vi "Test Queue Synch.vi"() -> ()   [LabVIEW 2021]
uses:
  Source/Support/Nodes/abs_Node/Status.ctl
  Source/System/bt_System.lvclass
  Source/Support/Nodes/Decorators/Repeater/Support/Finish On - Type.ctl
  Source/Support/Nodes/Composites/abs_Parallel/Support/Status Calculation.ctl
  Source/Blackboard/Blackboard.lvclass
  Source/Blackboard/Blackboard.lvclass/Blackboard.ctl
  Source/Support/Nodes/Leaves/abs_Type Leaf/abs_Type Leaf.lvclass/abs_Type Leaf.ctl
  Source/Blackboard/Get Value Type/Get Boolean.vi
  Source/Blackboard/Get Value Type/Get String.vi
  Source/Blackboard/Get Value Type/Get I32.vi
  <vilib>/TSA/Abstract Data Classes/Abs_Types/String/Static Read.vi
  <vilib>/TSA/Abstract Data Classes/Abs_Types/I32 Integer/Static Read.vi
  <vilib>/TSA/Abstract Data Classes/Abs_Types/Boolean/Static Read.vi
  Source/Blackboard/Support/Index Group.vi
  Source/Blackboard/Support/Index Tags.vi
  Source/Support/Nodes/Leaves/abs_Type Leaf/Properties/Write Value Class.vi
  <vilib>/TSA/Omni-Bus/Local Bus/Support/Bool/Local Bus_Boolean.lvclass
  C:/Program Files (x86)/National Instruments/LabVIEW 2021/vi.lib/TSA/Abstract Data Classes/Abs_Types/Value/Abs_Value.lvclass
  Source/Support/Nodes/Leaves/Test Boolean/Test Abs_Boolean.lvclass
  C:/Users/Tim/Documents/GitHub/LV_Behaviour_Tree/Source/Support/Nodes/abs_Node/bt_Node.lvclass
  C:/Users/Tim/Documents/GitHub/LV_Behaviour_Tree/Source/Support/Nodes/Leaves/abs_Type Leaf/abs_Type Leaf.lvclass
  <vilib>/TSA/Abstract Data Classes/Abs_Types/Boolean/Abs_Boolean.lvclass
  C:/Program Files (x86)/National Instruments/LabVIEW 2021/vi.lib/TSA/Abstract Data Classes/Abs_Types/Type/Abs_Type.lvclass
  <vilib>/TSA/Omni-Bus/Local Bus/Support/I32/Local Bus_I32.lvclass
  <vilib>/TSA/Omni-Bus/Local Bus/Support/STR/Local Bus_String.lvclass
  Source/Support/Nodes/Leaves/Synch/Queue/Send/bt_Send_Queue.lvclass
  Source/Support/Nodes/Leaves/Synch/Queue/WaitOn/bt_WaitOn_Queue.lvclass
  <vilib>/TSA/Omni-Bus/Local Bus/Support/Initialise DVR's.vi
  <vilib>/TSA/Abstract Data Classes/Abs_Types/Value/Abs_Value.lvclass
  <vilib>/TSA/Abstract Data Classes/Abs_Types/Type/Abs_Type.lvclass
  <vilib>/TSA/Omni-Bus/Local Bus/Support/DBL/Local Bus_DBL.lvclass
  <vilib>/TSA/Omni-Bus/Local Bus/Support/SGL/Local Bus_SGL.lvclass
  <vilib>/TSA/Omni-Bus/Local Bus/Support/EXT/Local Bus_EXT.lvclass
  <vilib>/TSA/Omni-Bus/Local Bus/Support/Variant/Local Bus_Variant.lvclass
  <vilib>/TSA/Omni-Bus/Local Bus/Support/WFM/Local Bus_Waveform.lvclass
  <vilib>/TSA/Omni-Bus/Local Bus/Support/Time/Local Bus_Time.lvclass
  <vilib>/TSA/Omni-Bus/Local Bus/Support/U8/Local Bus_U8.lvclass
  <vilib>/TSA/Omni-Bus/Local Bus/Support/U16/Local Bus_U16.lvclass
  <vilib>/TSA/Omni-Bus/Local Bus/Support/U32/Local Bus_U32.lvclass
  <vilib>/TSA/Omni-Bus/Local Bus/Support/U64/Local Bus_U64.lvclass
  <vilib>/TSA/Omni-Bus/Local Bus/Support/I8/Local Bus_I8.lvclass
  <vilib>/TSA/Omni-Bus/Local Bus/Support/I16/Local Bus_I16.lvclass
  <vilib>/TSA/Omni-Bus/Local Bus/Support/I64/Local Bus_I64.lvclass
  <vilib>/TSA/Omni-Bus/Local Bus/Support/CSGL/Local Bus_CSGL.lvclass
  <vilib>/TSA/Omni-Bus/Local Bus/Support/CDBL/Local Bus_CDBL.lvclass
  <vilib>/TSA/Omni-Bus/Local Bus/Support/CEXT/Local Bus_CEXT.lvclass
  <vilib>/TSA/Omni-Bus/Local Bus/Support/Type/Local Bus_Type.lvclass
  <vilib>/TSA/Abstract Data Classes/Abs_Types/I32 Integer/Abs_I32 Integer.lvclass
  <vilib>/TSA/Abstract Data Classes/Abs_Types/String/Abs_String.lvclass
  Source/BT.lvlib
  Source/Support/Nodes/Composites/abs_Parallel/bt_Parallel.lvclass
  Source/Support/Nodes/Decorators/Repeater/bt_Repeater.lvclass
  Source/Support/Nodes/abs_Node/bt_Node.lvclass
panel:
  out "error out 4":errorcluster
  out "error out 3":errorcluster
  out "error out 2":errorcluster
  out "error out":errorcluster
  out "String":string
  out "Value":i32
  out "Boolean":bool
  in  "stop":bool
  out "Status":T1
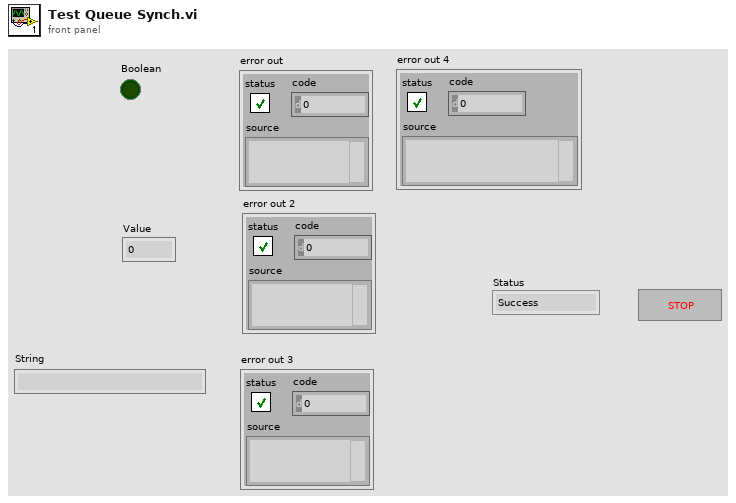
[diagram p1: front panel]
types:
  T1 = typedef "BT.lvlib/bt_Node.lvclass/Status.ctl" = enum16{"Success", "Failure", "Running"}
  T2 = typedef "BT.lvlib/bt_Parallel.lvclass/Status Calculation.ctl" = enum16{"Succeed on All Succeed", "Failure on All Failure", "Succeed on Any Succeed", "Failure on Any Failure"}
  T3 = typedef "BT.lvlib/bt_Repeater.lvclass/Finish On - Type.ctl" = enum16{"Success", "Failure", "Never"}
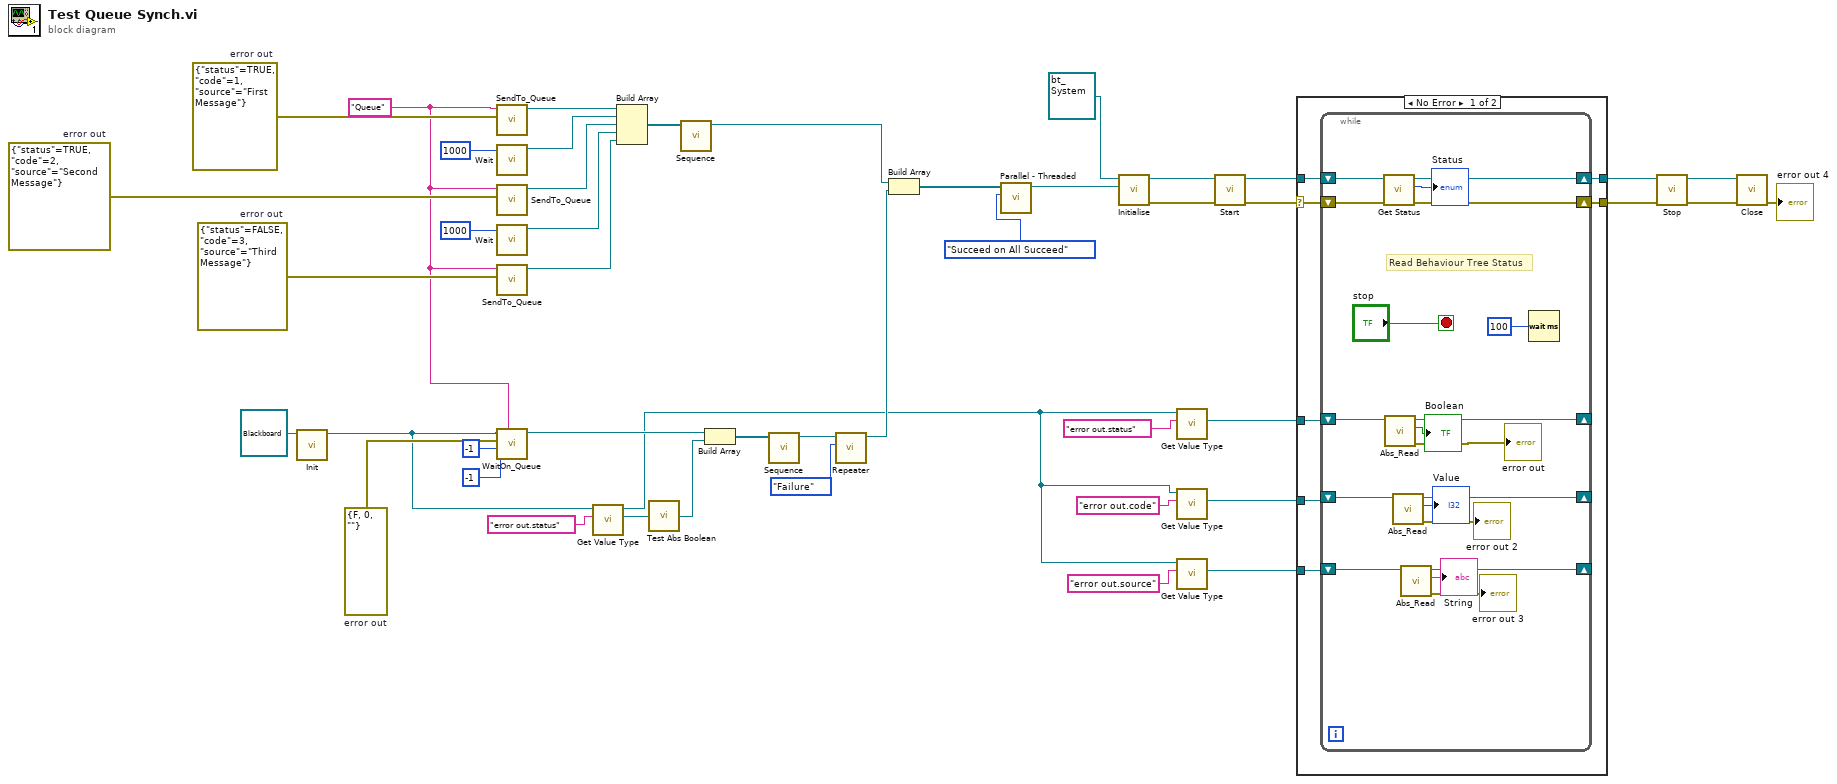
[diagram p0: block diagram]
diagram:
  w16 = errorcluster {"status"=FALSE, "code"=3, "source"="Third Message"}  # error out
  w18 = errorcluster {"status"=TRUE, "code"=2, "source"="Second Message"}  # error out
  w19 = errorcluster {"status"=TRUE, "code"=1, "source"="First Message"}  # error out
  w20 = errorcluster {"status"=FALSE, "code"=0, "source"=""}  # error out
  w6 = "Queue" ("Name")
  n1 = call-dynamic "Init.vi"("bt_Blackboard in"=refnum<class "Blackboard.lvclass"> refnum) -> ("bt_Blackboard out"=w11:refnum<class "Blackboard.lvclass">)  [unwired: 9 in, 1 out]
  n2 = call "SendTo_Queue.vi"("Message"=w19, "Queue Name"=w6) -> ("Queue Out"=w35:refnum<class "bt_Send_Queue.lvclass">)  [unwired: 9 in]
  n3 = call "Wait.vi"("Time (ms)"=u32 1000) -> ("Node Out"=w27:refnum<class "bt_Node.lvclass">)  [unwired: 10 in]
  n4 = call "SendTo_Queue.vi"("Message"=w18, "Queue Name"=w6) -> ("Queue Out"=w33:refnum<class "bt_Send_Queue.lvclass">)  [unwired: 9 in]
  n5 = call "Wait.vi"("Time (ms)"=u32 1000) -> ("Node Out"=w25:refnum<class "bt_Node.lvclass">)  [unwired: 10 in]
  n6 = call "SendTo_Queue.vi"("Message"=w16, "Queue Name"=w6) -> ("Queue Out"=w32:refnum<class "bt_Send_Queue.lvclass">)  [unwired: 9 in]
  n7 = call "WaitOn_Queue.vi"("Queue Name"=w6, "Max Queue Size"=-1, "Timeout (ms)"=-1, "Message Type"=w20, "bt_Blackboard in"=w11) -> ("Queue out"=w30:refnum<class "bt_WaitOn_Queue.lvclass">)  [unwired: 5 in, 1 out]
  n8 = call-poly "Get Value Type.vi"("Tag"="error out.status", "Blackboard in"=w11) -> ("Value"=w12:refnum<class "Abs_Boolean.lvclass">, "Blackboard out"=w5:refnum<class "Blackboard.lvclass">)  [unwired: 6 in, 2 out]
  n9 = Build Array(w35, w27, w33, w25, w32) -> (w34:refnum<class "bt_Node.lvclass">[])
  n10 = call "Test Abs Boolean.vi"("Abs_Boolean.lvclass"=w12) -> ("abs_Node"=w24:refnum<class "bt_Node.lvclass">)  [unwired: 4 in]
  n11 = call "Sequence.vi"("Nodes"=w34) -> ("Node"=w31:refnum<class "bt_Node.lvclass">)  [unwired: 10 in]
  n12 = Build Array(w30, w24) -> (w29:refnum<class "bt_Node.lvclass">[])
  n13 = call "Sequence.vi"("Nodes"=w29) -> ("Node"=w23:refnum<class "bt_Node.lvclass">)  [unwired: 10 in]
  n14 = call "Repeater.vi"("Finish On"=Finish_On_-_Type."Failure", "Node In"=w23) -> ("Node Out"=w21:refnum<class "bt_Node.lvclass">)  [unwired: 9 in]
  n15 = Build Array(w31, w21) -> (w37:refnum<class "bt_Node.lvclass">[])
  n16 = call "Parallel - Threaded.vi"("Status Calculation"=Status_Calculation."Succeed on All Succeed", "Nodes"=w37) -> ("Node"=w36:refnum<class "bt_Node.lvclass">)  [unwired: 9 in]
  n17 = call "Initialise.vi"("Behaviour Tree"=w36, "bt_System in"=refnum<class "bt_System.lvclass"> refnum) -> ("error out"=w45:errorcluster, "bt_System out"=w46:refnum<class "bt_System.lvclass">)  [unwired: 8 in]
  n18 = call-poly "Get Value Type.vi"("Tag"="error out.status", "Blackboard in"=w5) -> ("Value"=w14:refnum<class "Abs_Boolean.lvclass">)  [unwired: 6 in, 3 out]
  n19 = call-poly "Get Value Type.vi"("Tag"="error out.code", "Blackboard in"=w5) -> ("Value"=w8:refnum<class "Abs_I32 Integer.lvclass">)  [unwired: 6 in, 3 out]
  n20 = call-poly "Get Value Type.vi"("Tag"="error out.source", "Blackboard in"=w5) -> ("Value"=w4:refnum<class "Abs_String.lvclass">)  [unwired: 6 in, 3 out]
  n21 = call "Start.vi"("error in (no error)"=w45, "bt_System in"=w46) -> ("error out"=w3:errorcluster, "bt_System out"=w43:refnum<class "bt_System.lvclass">)  [unwired: 8 in]
  n22 = case shown="No Error" w3 {
    selector: w3 -> [w48 w73]
    tunnel: w43 -> [w53 w74]
    tunnel: [w52 w74] -> w40
    tunnel: w14 -> [w51 _]
    tunnel: w8 -> [w50 _]
    tunnel: w4 -> [w49 _]
    tunnel: [w47 w73] -> w2
    frame No Error {
      n23 = while {
        shift-right: [w70] -> w52
        shift-left: w53 -> [w71]
        shift-right: [w66] -> _
        shift-left: w51 -> [w67]
        shift-right: [w64] -> _
        shift-left: w50 -> [w65]
        shift-right: [w62] -> _
        shift-left: w49 -> [w63]
        shift-right: [w54] -> w47
        shift-left: w48 -> [w55]
        stop <- "stop" stop-if-true
        # "Read Behaviour Tree Status"
        n24 = call "Get Status.vi"("error in (no error)"=w55, "bt_System in"=w71) -> ("error out"=w54:errorcluster, "Status"=→"Status":T1, "bt_System out"=w70:refnum<class "bt_System.lvclass">)  [unwired: 7 in]
        n25 = call-poly <vilib>:"Abs_Read.vi"("Abs_Boolean in"=w67) -> ("error out"=→"error out":errorcluster, "Boolean"=→"Boolean":bool, "Abs_Boolean out"=w66:refnum<class "Abs_Boolean.lvclass">)  [unwired: 8 in]
        n26 = call-poly <vilib>:"Abs_Read.vi"("Abs_I32 Integer in"=w65) -> ("error out"=→"error out 2":errorcluster, "Value"=→"Value":i32, "Abs_I32 Integer out"=w64:refnum<class "Abs_I32 Integer.lvclass">)  [unwired: 8 in]
        n27 = call-poly <vilib>:"Abs_Read.vi"("Abs_String in"=w63) -> ("error out"=→"error out 3":errorcluster, "String"=→"String":string, "Abs_String out"=w62:refnum<class "Abs_String.lvclass">)  [unwired: 8 in]
        n28 = Wait (ms)(milliseconds to wait=u32 100) -> ()  [unwired: 1 out]
      }
    }
    frame Error {
    }
  }
  n29 = call "Stop.vi"("error in (no error)"=w2, "bt_System in"=w40) -> ("error out"=w41:errorcluster, "bt_System out"=w42:refnum<class "bt_System.lvclass">)  [unwired: 8 in]
  n30 = call-dynamic "Close.vi"("error in (no error)"=w41, "bt_System in"=w42) -> ("error out"=→"error out 4":errorcluster)  [unwired: 8 in, 1 out]
